vi "获取IP地址.vi"() -> (1 "名称":string)   [LabVIEW 2016, in "TCP发送文件.lvlib"]
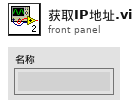
[diagram p1: front panel]
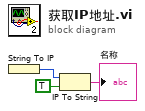
[diagram p0: block diagram]
diagram:
  n1 = String To IP() -> (0:w2:u32)  [unwired: 1 in]
  n2 = IP To String(1:TRUE ("句点符号？(F)"), 2:w2) -> (0:→"名称":string)
